vi "Stream Write Digital Outputs.vi"(7 "Digital Outputs":bool[](array[boolean]), 8 "error in (no error)":errorcluster, 9 "Device Number":string, 10 "Stream Number (1)":u8=1, 11 "VISA resource name":refnum<visa-resource-name>) -> (0 "error out":errorcluster, 3 "VISA resource name out":refnum<visa-resource-name>)   [LabVIEW 2013, in "Zaber A Series.lvlib"]
doc: "Writes to the digital output pins on a Zaber controller device such as the A-MCB or X-MCB series devices, as part of a streamed command sequence. Input is an array of booleans that must have the same number of elements as there are digital output pins on the device - use the Get I/O Pin Counts VI to determine this.\n \nThis VI requires that the Initialize VI has been called with the same serial port and that the specified stream has already been opened."
uses:
  Zaber A Series.lvlib
  Private/All Commands.ctl
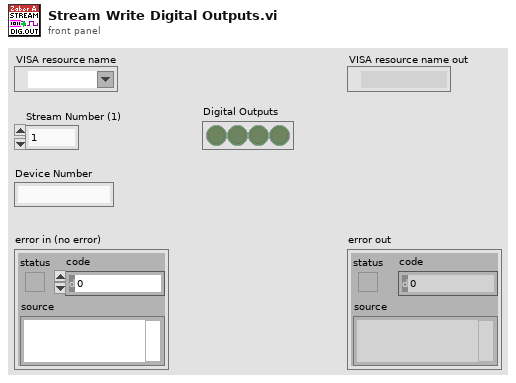
[diagram p1: front panel]
types:
  T1 = typedef "Zaber A Series.lvlib/All Commands.ctl" = string
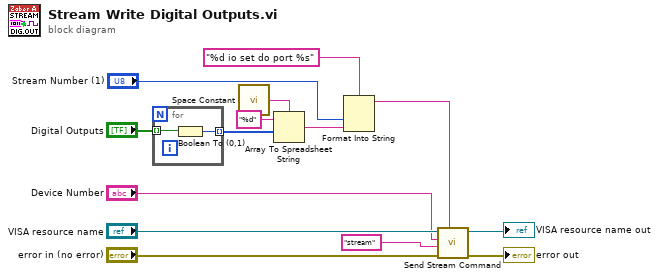
[diagram p0: block diagram]
diagram:
  n1 = for {
    tunnel: "Digital Outputs" -> [w16] mode=indexing
    tunnel: [w15] -> w13 mode=indexing
    n2 = Boolean To (0,1)(Boolean=w16) -> (0, 1=w15:i16)
  }
  n3 = call <vilib>:"Space Constant.vi"() -> ("String"=w11:string)
  n4 = Array To Spreadsheet String(delimiter (Tab)=w11, array=w13, 3:"%d" ("format string")) -> (spreadsheet string=w3:string)
  n5 = Format Into String(format string="%d io set do port %s", "Stream Number (1)", w3) -> (resulting string=w2:string)  [unwired: 2 in, 1 out]
  n6 = call "Send Stream Command.vi"("Data"=w2, "error in (no error)"="error in (no error)", "Command"=T1 "stream" ("Complete Command List"), "Device Number"="Device Number", "VISA resource name"="VISA resource name") -> ("error out"=→"error out":errorcluster, "VISA resource name out"=→"VISA resource name out":refnum<visa-resource-name>)  [unwired: 5 in]
